vi "Acknowledgement.vi"(5 "Ack Comm":T1, 6 "Inc":bool, 7 "Numeric":i32=75, 8 "error in (no error)":errorcluster, 11 "VISA resource name":refnum<visa-resource-name>) -> (0 "error out":errorcluster, 2 "Connected?":bool, 3 "VISA resource name out":refnum<visa-resource-name>)   [LabVIEW 2018]
uses:
  Controls/ACK Comm.ctl
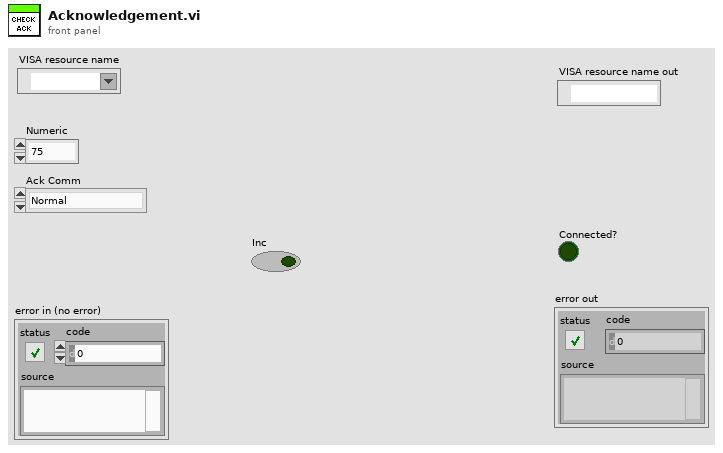
[diagram p1: front panel]
types:
  T1 = typedef "ACK Comm.ctl" = enum16{"Normal", "Filter Selection", "Shuuter Open", "Shutter Close"}
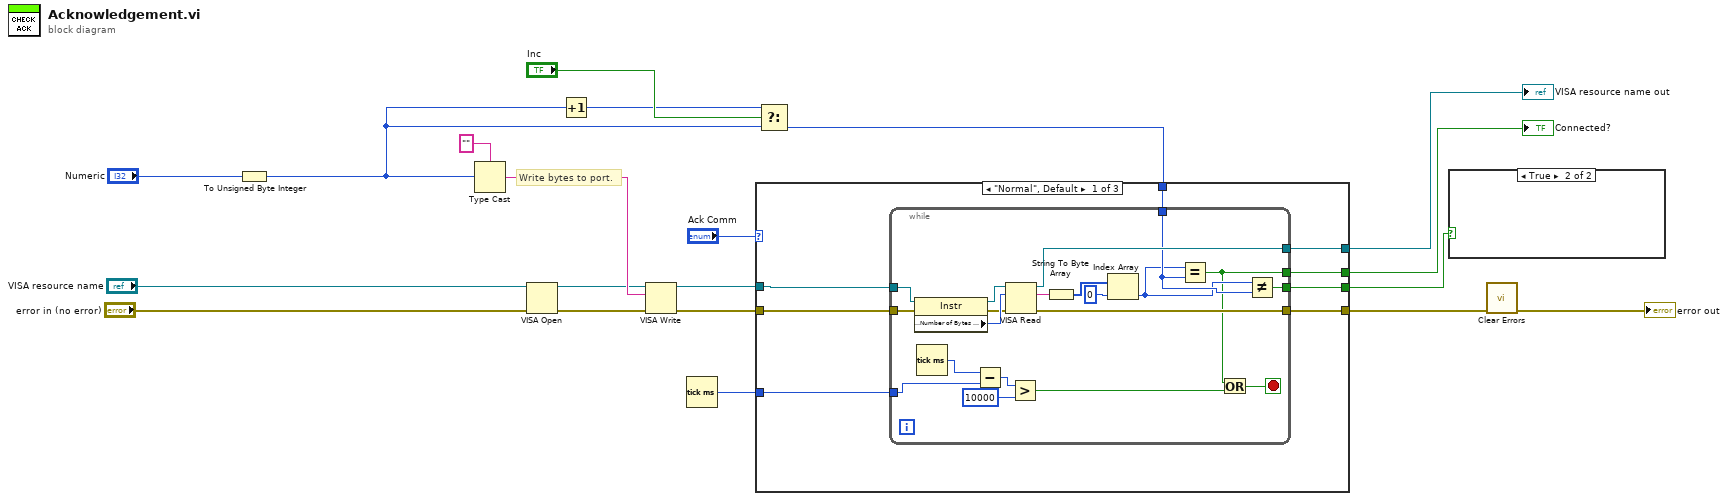
[diagram p0: block diagram]
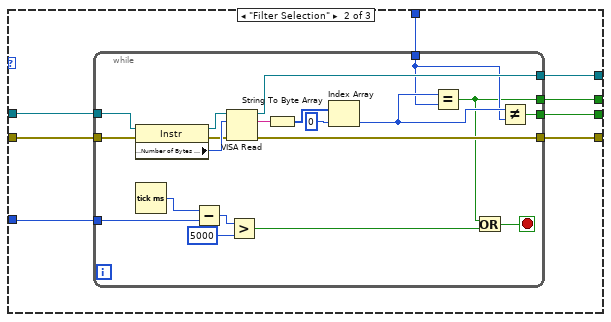
[diagram p2: hidden frame]
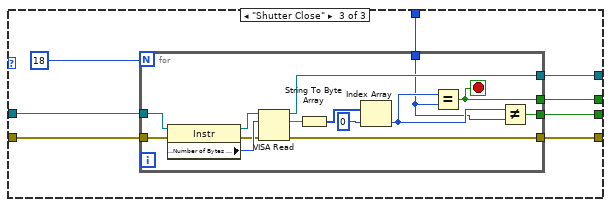
[diagram p3: hidden frame]
diagram:
  # "Write bytes to port."
  n1 = To Unsigned Byte Integer(number="Numeric") -> (unsigned 8bit integer=w2:u8)
  n2 = Type Cast(type="", x=w2) -> (*(type *) &x=w15:string)
  n3 = VISA Open(error in (no error)="error in (no error)", VISA resource name="VISA resource name") -> (VISA resource name=w14:refnum<visa-resource-name>, error out=w13:errorcluster)  [unwired: 3 in]
  n4 = Increment(x=w2) -> (x+1=w1:u8)
  n5 = VISA Write(VISA resource name=w14, write buffer=w15, error in (no error)=w13) -> (VISA resource name out=w16:refnum<visa-resource-name>, error out=w5:errorcluster)  [unwired: 1 out]
  n6 = Tick Count (ms)() -> (millisecond timer value=w6:u32)
  n7 = Select(t=w1, s="Inc", f=w2) -> (s? t:f=w4:u8)
  n8 = case shown="\"Normal\", Default" "Ack Comm" {
    tunnel: [w28 w56 w84] -> w18
    tunnel: [w27 w55 w83] -> w17
    tunnel: w5 -> [w26 w54 w82]
    tunnel: w16 -> [w25 w53 w81]
    tunnel: [w24 w52 w79] -> w11
    tunnel: [w23 w51 w78] -> w10
    tunnel: w4 -> [w22 w50 w77]
    tunnel: w6 -> [w21 w49 _]
    frame "Normal", Default {
      n9 = while {
        tunnel: [w48] -> w28
        tunnel: [w35] -> w27
        tunnel: w22 -> [w44]
        tunnel: w25 -> [w47]
        tunnel: [w45] -> w23
        tunnel: w26 -> [w43]
        tunnel: [w46] -> w24
        tunnel: w21 -> [w29]
        stop <- w31 stop-if-true
        n10 = property class="Instr"(reference=w47, error in=w43) -> (reference out=w39:refnum<visa-resource-name>, error out=w37:errorcluster, "Serial Settings:Number of Bytes at Serial Port"=w38:u32)
        n11 = Tick Count (ms)() -> (millisecond timer value=w34:u32)
        n12 = Subtract(x=w34, y=w29) -> (x-y=w33:u32)
        n13 = VISA Read(VISA resource name=w39, byte count=w38, error in (no error)=w37) -> (VISA resource name out=w45:refnum<visa-resource-name>, read buffer=w42:string, error out=w46:errorcluster)  [unwired: 1 out]
        n14 = Greater?(x=w33, y=u32 10000) -> (0:w30:bool)
        n15 = String To Byte Array(string=w42) -> (unsigned byte array=w41:u8[])
        n16 = Index Array(array=w41, index=0) -> (element=w36:u8)
        n17 = Equal?(x=w36, y=w44) -> (x = y?=w35:bool)
        n18 = Or(x=w35, y=w30) -> (x .or. y?=w31:bool)
        n19 = Not Equal?(x=w36, y=w44) -> (x != y?=w48:bool)
      }
    }
    frame "Filter Selection" {
      n20 = while {
        tunnel: w53 -> [w70]
        tunnel: w54 -> [w71]
        tunnel: [w73] -> w51
        tunnel: [w72] -> w52
        tunnel: [w57] -> w55
        tunnel: [w65] -> w56
        tunnel: w50 -> [w64]
        tunnel: w49 -> [w60]
        stop <- w59 stop-if-true
        n21 = property class="Instr"(reference=w70, error in=w71) -> (reference out=w69:refnum<visa-resource-name>, error out=w67:errorcluster, "Serial Settings:Number of Bytes at Serial Port"=w68:u32)
        n22 = Tick Count (ms)() -> (millisecond timer value=w63:u32)
        n23 = Subtract(x=w63, y=w60) -> (x-y=w62:u32)
        n24 = VISA Read(VISA resource name=w69, byte count=w68, error in (no error)=w67) -> (VISA resource name out=w73:refnum<visa-resource-name>, read buffer=w76:string, error out=w72:errorcluster)  [unwired: 1 out]
        n25 = Greater?(x=w62, y=u32 5000) -> (0:w58:bool)
        n26 = String To Byte Array(string=w76) -> (unsigned byte array=w75:u8[])
        n27 = Index Array(array=w75, index=0) -> (element=w66:u8)
        n28 = Equal?(x=w66, y=w64) -> (x = y?=w57:bool)
        n29 = Or(x=w57, y=w58) -> (x .or. y?=w59:bool)
        n30 = Not Equal?(x=w66, y=w64) -> (x != y?=w65:bool)
      }
    }
    frame "Shutter Close" {
      n31 = for {
        N: 18 -> [_]
        tunnel: w81 -> [w92]
        tunnel: w82 -> [w93]
        tunnel: [w95] -> w78
        tunnel: [w94] -> w79
        tunnel: [w88] -> w83
        tunnel: [w86] -> w84
        tunnel: w77 -> [w85]
        stop <- w88 stop-if-true
        n32 = property class="Instr"(reference=w92, error in=w93) -> (reference out=w91:refnum<visa-resource-name>, error out=w89:errorcluster, "Serial Settings:Number of Bytes at Serial Port"=w90:u32)
        n33 = VISA Read(VISA resource name=w91, byte count=w90, error in (no error)=w89) -> (VISA resource name out=w95:refnum<visa-resource-name>, read buffer=w98:string, error out=w94:errorcluster)  [unwired: 1 out]
        n34 = String To Byte Array(string=w98) -> (unsigned byte array=w97:u8[])
        n35 = Index Array(array=w97, index=0) -> (element=w87:u8)
        n36 = Equal?(x=w87, y=w85) -> (x = y?=w88:bool)
        n37 = Not Equal?(x=w87, y=w85) -> (x != y?=w86:bool)
      }
    }
  }
  "Connected?" <- w17
  "VISA resource name out" <- w10
  n38 = case shown="True" w18 {
    frame False {
    }
    frame True {
    }
  }
  n39 = call <vilib>:"Clear Errors.vi"("error in (no error)"=w11) -> ("error out"=→"error out":errorcluster)  [unwired: 5 in, 1 out]
